vi "closeoptiMOS.vi"(6 "error in (no error)":errorcluster, 9 "Camera Handle":u32) -> (0 "error out":errorcluster)   [LabVIEW 2015]
uses:
  LabVIEW/Examples2014_4_3_2_7/Fast Examples/Open-Close Hardware/CamHandle.vi
panel:
  out "Camera close":bool
  # "ExCloseGlobalCam: this subvi closes a camera that uses the gloabal\ncamera handle."
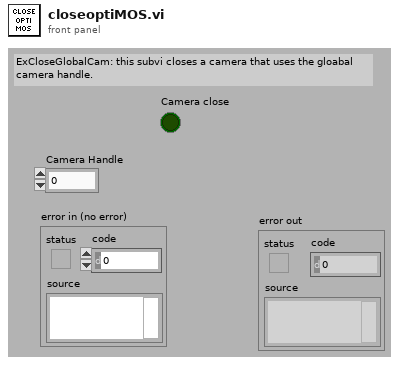
[diagram p1: front panel]
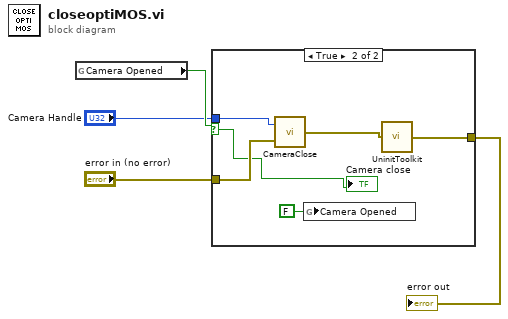
[diagram p0: block diagram]
diagram:
  n1 = global read "CamHandle.vi" "Camera Opened"() -> (w4:bool)
  n2 = case shown="True" w4 {
    selector: w4 -> [_ w8]
    tunnel: "error in (no error)" -> [w5 w11]
    tunnel: [w5 w9] -> w2
    tunnel: "Camera Handle" -> [_ w7]
    frame False {
    }
    frame True {
      n3 = call <userlib>:"CameraClose.vi"("error in"=w11, "Camera Handle"=w7) -> ("error out"=w10:errorcluster)
      n4 = global write "CamHandle.vi" "Camera Opened"(FALSE ("Camera Opened")) -> ()
      n5 = call <userlib>:"UninitToolkit.vi"("error in"=w10) -> ("error out"=w9:errorcluster)
      "Camera close" <- w8
    }
  }
  "error out" <- w2
